vi "Measurement Logic.vi"() -> ()   [LabVIEW 2020, in "NIDCPowerSourceDCVoltage.lvlib"]
uses:
  NIDCPowerSourceDCVoltage.lvlib
  Measurement Configuration.ctl
  Measurement Results.ctl
  <vilib>/MeasurementLink/MeasurementLink Measurement Server/Classes/MeasurementContext/MeasurementContext.lvclass
  <vilib>/MeasurementLink/MeasurementLink Discovery Client/RPC Messages/ni_measurementlink_discovery_v1_ResolveServiceRequest.ctl
  <vilib>/MeasurementLink/MeasurementLink Session Management Client/RPC Messages/ni_measurementlink_sessionmanagement_v1_ReserveSessionsRequest.ctl
  <vilib>/MeasurementLink/MeasurementLink Session Management Client/RPC Messages/ni_measurementlink_PinMapContext.ctl
  <vilib>/MeasurementLink/MeasurementLink Discovery Client/MeasurementLink Discovery Client.lvlib
  <vilib>/MeasurementLink/MeasurementLink Measurement Server/MeasurementLink Measurement Server.lvlib
  <vilib>/MeasurementLink/MeasurementLink Session Management Client/MeasurementLink Session Management Client.lvlib
panel:
  out "Measurement Context out":refnum<class "MeasurementContext.lvclass">
  in  "Measurement Context":refnum<class "MeasurementContext.lvclass">
  out "Measurement Results":T1
  in  "Measurement Configuration":T2={"pin_names"=[], "voltage_level"=6.0, "voltage_level_range"=6.0, "current_limit"=0.01, "current_limit_range"=0.01, "source_delay"=0.0}
  out "error out":errorcluster
  in  "error in":errorcluster
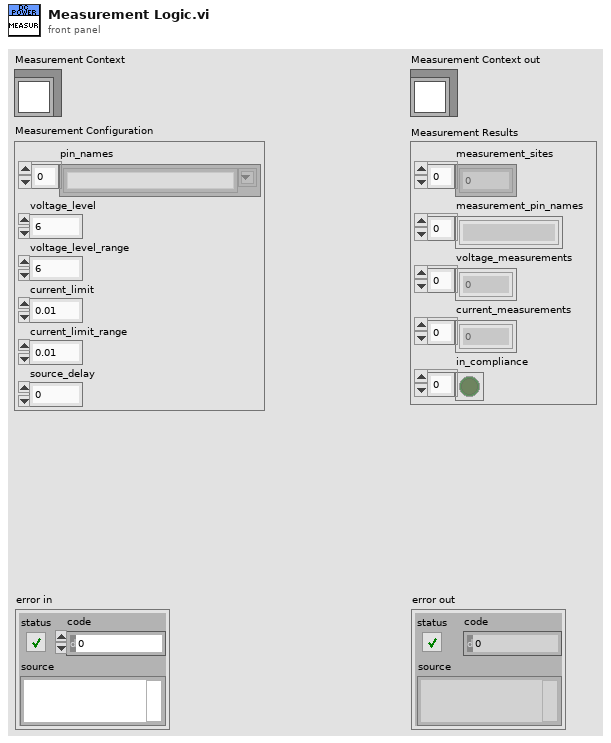
[diagram p1: front panel]
types:
  T1 = typedef "NIDCPowerSourceDCVoltage.lvlib/Measurement Results.ctl" = cluster{"measurement_sites":i32[], "measurement_pin_names":string[], "voltage_measurements":dbl[], "current_measurements":dbl[], "in_compliance":bool[]}
  T2 = typedef "NIDCPowerSourceDCVoltage.lvlib/Measurement Configuration.ctl" = cluster{"pin_names":string[], "voltage_level":dbl, "voltage_level_range":dbl, "current_limit":dbl, "current_limit_range":dbl, "source_delay":dbl}
  T3 = typedef "MeasurementLink Discovery Client.lvlib/ni_measurementlink_discovery_v1_ResolveServiceRequest.ctl" = cluster{"provided_interface":string, "service_class":string}
  T4 = typedef "MeasurementLink Session Management Client.lvlib/ni_measurementlink_sessionmanagement_v1_ReserveSessionsRequest.ctl" = cluster{"pin_map_context":T5, "pin_or_relay_names":string[], "instrument_type_id":string, "timeout_in_milliseconds":i32}
  T5 = typedef "MeasurementLink Session Management Client.lvlib/ni_measurementlink_PinMapContext.ctl" = cluster{"pin_map_id":string, "sites":i32[]}
  T6 = typedef "MeasurementLink Measurement Server Internal.lvlib/ni_measurementlink_PinMapContext.ctl" = cluster{"pin_map_id":string, "sites":i32[]}
  T7 = typedef "grpc-lvsupport-release.lvlib/grpcId.ctl" = u64
  T8 = typedef "MeasurementLink Discovery Client.lvlib/ni_measurementlink_discovery_v1_ServiceLocation.ctl" = cluster{"location":string, "insecure_port":string, "ssl_authenticated_port":string}
  T9 = typedef "MeasurementLink Session Management Client.lvlib/ni_measurementlink_sessionmanagement_v1_ReserveSessionsResponse.ctl" = cluster{"sessions":T10[]}
  T10 = typedef "MeasurementLink Session Management Client.lvlib/ni_measurementlink_sessionmanagement_v1_SessionInformation.ctl" = cluster{"session":T11, "resource_name":string, "channel_list":string, "instrument_type_id":string, "session_exists":bool, "channel_mappings":T12[]}
  T11 = typedef "MeasurementLink Session Management Client.lvlib/nidevice_grpc_Session.ctl" = cluster{"name":string}
  T12 = typedef "MeasurementLink Session Management Client.lvlib/ni_measurementlink_sessionmanagement_v1_ChannelMapping.ctl" = cluster{"pin_or_relay_name":string, "site":i32, "channel":string}
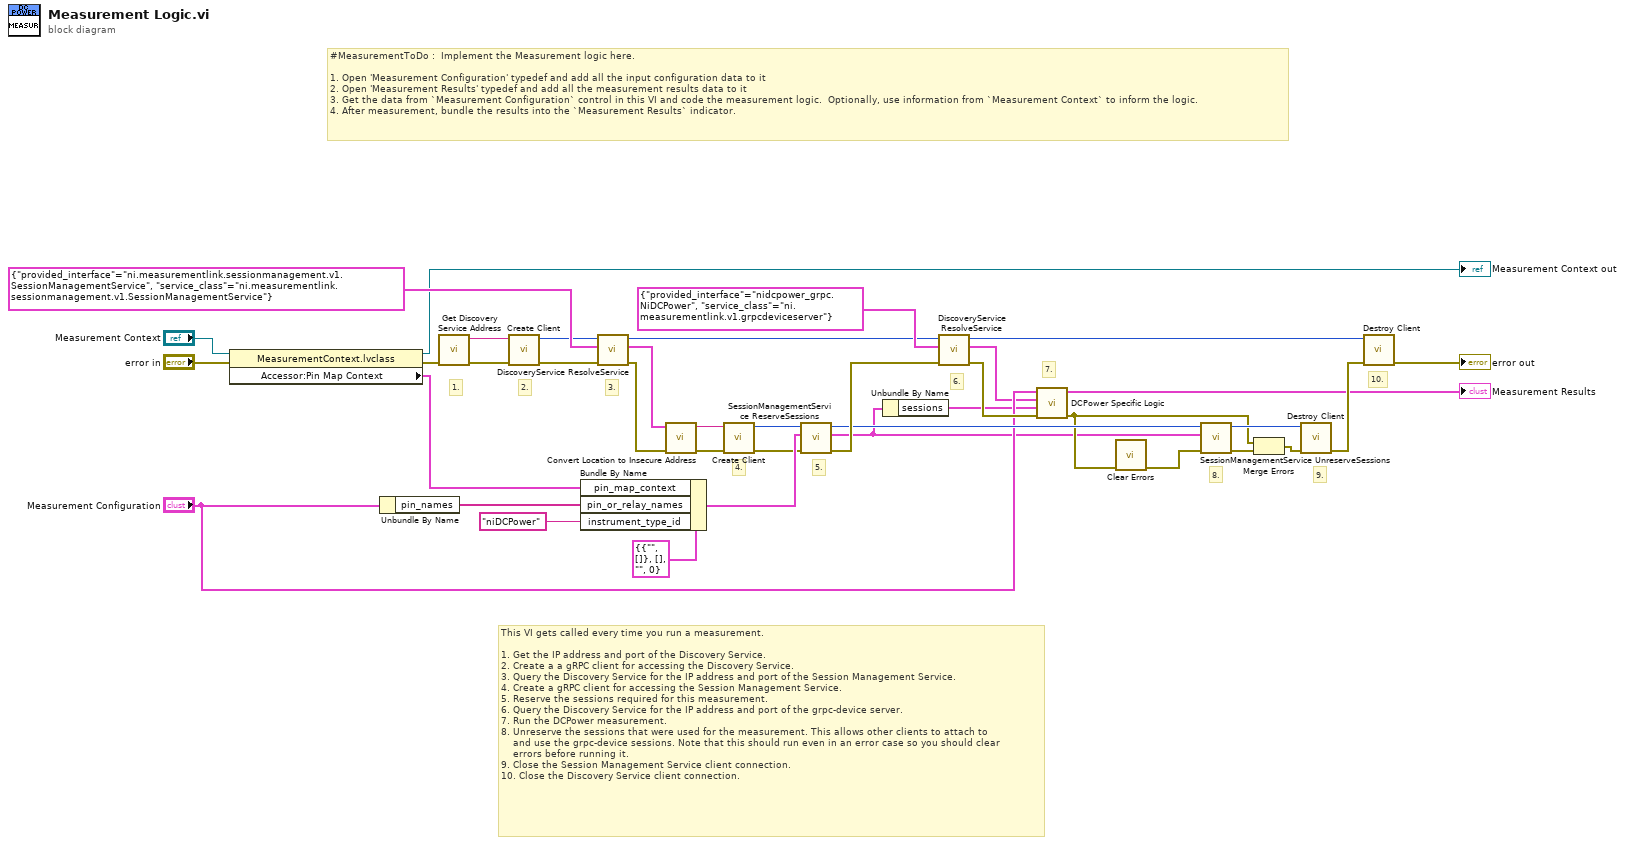
[diagram p0: block diagram]
diagram:
  # "10."
  # "9."
  # "8."
  # "7."
  # "6."
  # "5."
  # "4."
  # "3."
  # "2."
  # "This VI gets called every time you run a measurement.\n\n1. Get the IP address and port of the Discovery Service.\n2. Create a a gRPC client for accessing the Discovery Service.\n3. Query the Discovery Service for the IP address and port of the Session Management Service.\n4. Create a gRPC client for accessing the Session Management Service.\n5. Reserve the sessions required for this measurement.  \n6. Query the Discovery Service for the IP address and port of the grpc-device server.\n7. Run the DCPower measurement.\n8. Unreserve the sessions that were used for the measurement. This allows other clients to attach to\n    and use the grpc-device sessions. Note that this should run even in an error case so you should clear \n    errors before running it.\n9. Close the Session Management Service client connection.\n10. Close the Discovery Service client connection."
  # "1."
  # "#MeasurementToDo :  Implement the Measurement logic here.\n\n1. Open 'Measurement Configuration' typedef and add all the input configuration data to it\n2. Open 'Measurement Results' typedef and add all the measurement results data to it\n3. Get the data from `Measurement Configuration` control in this VI and code the measurement logic.  Optionally, use information from `Measurement Context` to inform the logic.\n4. After measurement, bundle the results into the `Measurement Results` indicator."
  n1 = property class="MeasurementContext.lvclass"(reference="Measurement Context", error in="error in") -> (reference out=→"Measurement Context out":refnum<class "MeasurementContext.lvclass">, error out=w5:errorcluster, "Accessor:Pin Map Context"=w2:T6)
  n2 = Unbundle By Name("Measurement Configuration") -> ("pin_names"=w26:string[])
  n3 = call <vilib>:"Get Discovery Service Address.vi"("error in"=w5) -> ("error out"=w37:errorcluster, "address"=w36:string)  [unwired: 9 in]
  n4 = call <vilib>:"Create Client.vi"("error in"=w37, "address"=w36) -> ("error out"=w27:errorcluster, "gRPC ID Out"=w31:T7)  [unwired: 8 in]
  n5 = Bundle By Name(cluster=T4 {"pin_map_context"={"pin_map_id"="", "sites"=[]}, "pin_or_relay_names"=[], "instrument_type_id"="", "timeout_in_milliseconds"=0} ("Request Data"), "pin_map_context"=w2, "pin_or_relay_names"=w26, "instrument_type_id"="niDCPower" ("Instrument Type Id")) -> (w28:T4)
  n6 = call <vilib>:"DiscoveryService ResolveService.vi"("error in"=w27, "Request Data"=T3 {"provided_interface"="ni.measurementlink.sessionmanagement.v1.SessionManagementService", "service_class"="ni.measurementlink.sessionmanagement.v1.SessionManagementService"}, "gRPC ID"=w31) -> ("error out"=w33:errorcluster, "Response Data"=w34:T8, "gRPC ID out"=w22:T7)  [unwired: 6 in]
  n7 = call "Convert Location to Insecure Address.vi"("Response Data"=w34) -> ("String"=w32:string)  [unwired: 10 in]
  n8 = call <vilib>:"Create Client.vi"("error in"=w33, "address"=w32) -> ("error out"=w1:errorcluster, "gRPC ID Out"=w30:T7)  [unwired: 8 in]
  n9 = call <vilib>:"SessionManagementService ReserveSessions.vi"("error in"=w1, "Request Data"=w28, "gRPC ID"=w30) -> ("error out"=w23:errorcluster, "Response Data"=w9:T9, "gRPC ID out"=w21:T7)  [unwired: 6 in]
  n10 = Unbundle By Name(w9) -> ("sessions"=w8:T10[])
  n11 = call <vilib>:"DiscoveryService ResolveService.vi"("error in"=w23, "Request Data"=T3 {"provided_interface"="nidcpower_grpc.NiDCPower", "service_class"="ni.measurementlink.v1.grpcdeviceserver"}, "gRPC ID"=w22) -> ("error out"=w13:errorcluster, "Response Data"=w10:T8, "gRPC ID out"=w18:T7)  [unwired: 6 in]
  n12 = call "DCPower Specific Logic.vi"("error in"=w13, "sessions"=w8, "Grpc Device Location"=w10, "Measurement Configuration"="Measurement Configuration") -> ("error out"=w12:errorcluster, "Measurement Results"=→"Measurement Results":T1)  [unwired: 6 in]
  n13 = call <vilib>:"Clear Errors.vi"("error in (no error)"=w12) -> ("error out"=w14:errorcluster)  [unwired: 5 in, 1 out]
  n14 = call <vilib>:"SessionManagementService UnreserveSessions.vi"("error in"=w14, "Request Data"=w9, "gRPC ID"=w21) -> ("error out"=w16:errorcluster, "gRPC ID out"=w20:T7)  [unwired: 6 in, 1 out]
  n15 = Merge Errors(w12, w16) -> (w15:errorcluster)
  n16 = call <vilib>:"Destroy Client.vi"("error in"=w15, "gRPC ID"=w20) -> ("error out"=w19:errorcluster)  [unwired: 9 in]
  n17 = call <vilib>:"Destroy Client.vi"("error in"=w19, "gRPC ID"=w18) -> ("error out"=→"error out":errorcluster)  [unwired: 9 in]
